vi "Envelop detect.vi"(8 "error in":errorcluster, 11 "Data in":dbl[](array[numeric])) -> (0 "error out":errorcluster, 3 "Envelop":dbl[](array[numeric]))   [LabVIEW 2016]
uses:
  <vilib>/Analysis/NI_AALPro.lvlib
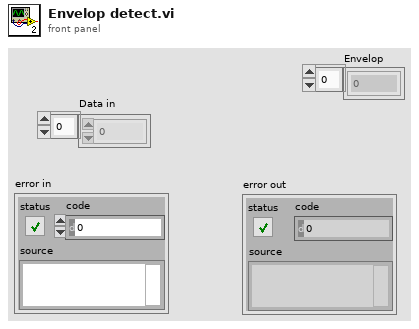
[diagram p1: front panel]
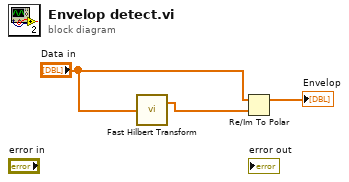
[diagram p0: block diagram]
diagram:
  n1 = call <vilib>:"Fast Hilbert Transform.vi"("X"="Data in") -> ("Hilbert{X}"=w3:dbl[])  [unwired: 1 out]
  n2 = Re/Im To Polar(2:w3, 3:"Data in") -> (1:→"Envelop":dbl[])  [unwired: 1 out]
